vi "createColorImFromU32arr.vi"(6 "max vals (-1 for autoscale)":cluster{"r max":dbl, "g max":dbl, "b max":dbl}={"r max"=-1.0, "g max"=-1.0, "b max"=-1.0}, 7 "b buffer":u32[][](array[numeric]), 8 "error in (no error)":errorcluster, 9 "g buffer":u32[][](array[numeric]), 10 "r buffer":u32[][](array[numeric]), 11 "Image":T1) -> (0 "error out":errorcluster, 2 "max vals from im":cluster{"r max":u32, "g max":u32, "b max":u32}, 3 "Image Out":T1)   [LabVIEW 2010]
uses:
  <vilib>/vision/Image Controls.llb/IMAQ Image.ctl
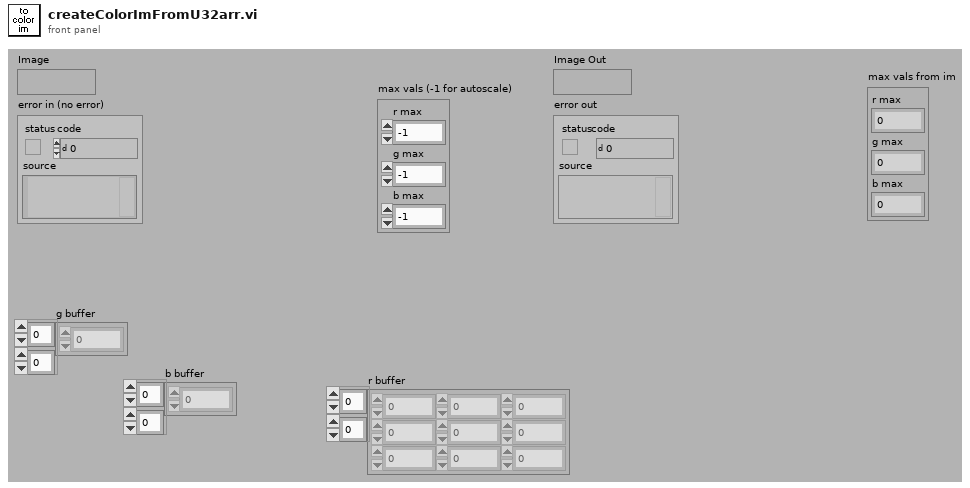
[diagram p1: front panel]
types:
  T1 = typedef "IMAQ Image.ctl" = refnum<image>
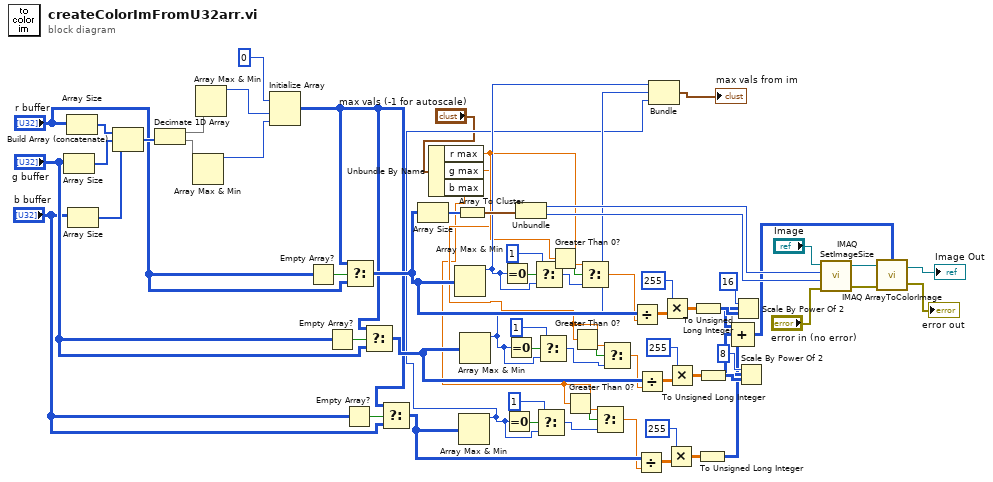
[diagram p0: block diagram]
diagram:
  n1 = Array Size(array="g buffer") -> (size(s)=w41:i32[])
  n2 = Array Size(array="r buffer") -> (size(s)=w42:i32[])
  n3 = Array Size(array="b buffer") -> (size(s)=w40:i32[])
  n4 = Build Array (concatenate)(w42, w41, w40) -> (w39:i32[])
  n5 = Decimate 1D Array(w39) -> (w38:i32[], w37:i32[])
  n6 = Array Max & Min(array=w37) -> (max value=w34:i32)  [unwired: 3 out]
  n7 = Array Max & Min(array=w38) -> (max value=w35:i32)  [unwired: 3 out]
  n8 = Initialize Array(u32 0, w35, w34) -> (w27:u32[][])
  n9 = Empty Array?(array="r buffer") -> (empty?=w33:bool)
  n10 = Empty Array?(array="g buffer") -> (empty?=w31:bool)
  n11 = Empty Array?(array="b buffer") -> (empty?=w29:bool)
  n12 = Select(t=w27, s=w33, f="r buffer") -> (s? t:f=w32:u32[][])
  n13 = Select(t=w27, s=w31, f="g buffer") -> (s? t:f=w30:u32[][])
  n14 = Select(t=w27, s=w29, f="b buffer") -> (s? t:f=w28:u32[][])
  n15 = Array Size(array=w32) -> (size(s)=w52:i32[])
  n16 = Unbundle By Name("max vals (-1 for autoscale)") -> ("r max"=w9:dbl, "g max"=w6:dbl, "b max"=w2:dbl)
  n17 = Array Max & Min(array=w32) -> (max value=w17:u32)  [unwired: 3 out]
  n18 = Array To Cluster(array=w52) -> (cluster=w51:cluster{"[0]":i32, "[1]":i32})
  n19 = Array Max & Min(array=w28) -> (max value=w15:u32)  [unwired: 3 out]
  n20 = Array Max & Min(array=w30) -> (max value=w16:u32)  [unwired: 3 out]
  n21 = Equal To 0?(x=w17) -> (x = 0?=w19:bool)
  n22 = Equal To 0?(x=w15) -> (x = 0?=w23:bool)
  n23 = Equal To 0?(x=w16) -> (x = 0?=w21:bool)
  n24 = Unbundle(w51) -> ("[0]"=w50:i32, "[1]"=w49:i32)
  n25 = Select(t=u32 1, s=w19, f=w17) -> (s? t:f=w11:u32)
  n26 = Select(t=u32 1, s=w23, f=w15) -> (s? t:f=w3:u32)
  n27 = Select(t=u32 1, s=w21, f=w16) -> (s? t:f=w7:u32)
  n28 = Greater Than 0?(x=w9) -> (x > 0?=w10:bool)
  n29 = Greater Than 0?(x=w2) -> (x > 0?=w4:bool)
  n30 = Greater Than 0?(x=w6) -> (x > 0?=w8:bool)
  n31 = Select(t=w9, s=w10, f=w11) -> (s? t:f=w12:dbl)
  n32 = Select(t=w2, s=w4, f=w3) -> (s? t:f=w1:dbl)
  n33 = Select(t=w6, s=w8, f=w7) -> (s? t:f=w5:dbl)
  n34 = Divide(x=w32, y=w12) -> (x/y=w69:dbl[][])
  n35 = Divide(x=w28, y=w1) -> (x/y=w63:dbl[][])
  n36 = Divide(x=w30, y=w5) -> (x/y=w66:dbl[][])
  n37 = Bundle(w17, w16, w15) -> (→"max vals from im":cluster{u32, u32, u32})  [unwired: 1 in]
  n38 = Multiply(x=255, y=w69) -> (x*y=w67:dbl[][])
  n39 = Multiply(x=255, y=w63) -> (x*y=w61:dbl[][])
  n40 = Multiply(x=255, y=w66) -> (x*y=w64:dbl[][])
  n41 = To Unsigned Long Integer(number=w67) -> (unsigned 32bit integer=w60:u32[][])
  n42 = To Unsigned Long Integer(number=w61) -> (unsigned 32bit integer=w54:u32[][])
  n43 = To Unsigned Long Integer(number=w64) -> (unsigned 32bit integer=w58:u32[][])
  n44 = Scale By Power Of 2(n=16, x=w60) -> (x*2^n=w56:u32[][])
  n45 = Scale By Power Of 2(n=8, x=w58) -> (x*2^n=w55:u32[][])
  n46 = Compound Arithmetic op=ADD(w56, w55, w54) -> (w45:u32[][])
  n47 = call "IMAQ SetImageSize"("error in (no error)"="error in (no error)", "Y Resolution"=w49, "X Resolution"=w50, "Image"="Image") -> ("error out"=w46:errorcluster, "Image Out"=w47:T1)  [unwired: 1 in]
  n48 = call "IMAQ ArrayToColorImage"("Image Pixels (U32)"=w45, "Image"=w47, "error in (no error)"=w46) -> ("Image Out"=→"Image Out":T1, "error out"=→"error out":errorcluster)  [unwired: 2 in]
